vi "floor selecter.vi"(5 "floor in":dbl, 8 "up/down in":T2) -> (0 "floor out":dbl, 1 "state":T1, 2 "T/F":bool, 3 "up/down out":T2)   [LabVIEW 2020]
uses:
  state.ctl
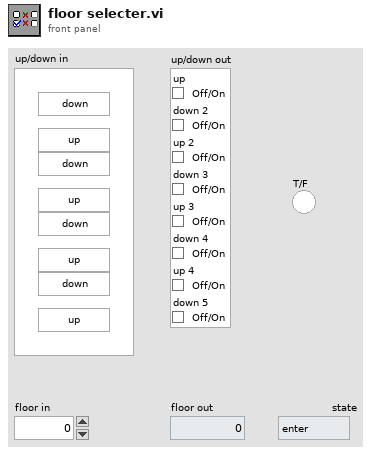
[diagram p1: front panel]
types:
  T1 = typedef "state.ctl" = enum16{"enter", "checking", "go up", "go down", "process", "get out", "temp"}
  T2 = cluster{"up":bool, "down 2":bool, "up 2":bool, "down 3":bool, "up 3":bool, "down 4":bool, "up 4":bool, "down 5":bool}
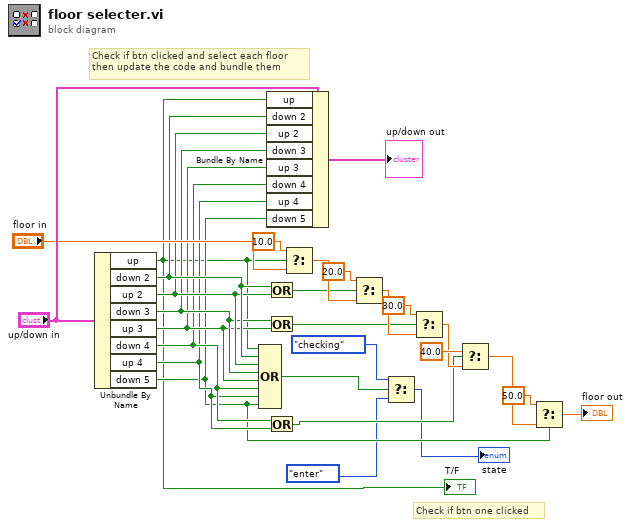
[diagram p0: block diagram]
diagram:
  # "Check if btn one clicked"
  # "Check if btn clicked and select each floor\nthen update the code and bundle them"
  n1 = Unbundle By Name("up/down in") -> ("up"=w1:bool, "down 2"=w12:bool, "up 2"=w11:bool, "down 3"=w10:bool, "up 3"=w9:bool, "down 4"=w8:bool, "up 4"=w7:bool, "down 5"=w6:bool)
  "T/F" <- w1
  n2 = Compound Arithmetic op=OR(w1, w12, w11, w10, w9, w8, w7, w6) -> (w2:bool)
  n3 = Bundle By Name(cluster="up/down in", "up"=w1, "down 2"=w12, "up 2"=w11, "down 3"=w10, "up 3"=w9, "down 4"=w8, "up 4"=w7, "down 5"=w6) -> (→"up/down out":T2)
  n4 = Or(x=w12, y=w11) -> (x .or. y?=w15:bool)
  n5 = Or(x=w10, y=w9) -> (x .or. y?=w16:bool)
  n6 = Or(x=w8, y=w7) -> (x .or. y?=w17:bool)
  n7 = Select(t=10.0, s=w1, f="floor in") -> (s? t:f=w18:dbl)
  n8 = Select(t=20.0, s=w15, f=w18) -> (s? t:f=w19:dbl)
  n9 = Select(t=state."checking", s=w2, f=state."enter") -> (s? t:f=→"state":T1)
  n10 = Select(t=30.0, s=w16, f=w19) -> (s? t:f=w20:dbl)
  n11 = Select(t=40.0, s=w17, f=w20) -> (s? t:f=w21:dbl)
  n12 = Select(t=50.0, s=w6, f=w21) -> (s? t:f=→"floor out":dbl)
